vi "K6514_VISAQuery.vi"() -> ()   [LabVIEW 2024]
panel:
  out "read buffer":string
  in  "write buffer":string
  in  "VISA resource name":refnum<visa-resource-name>
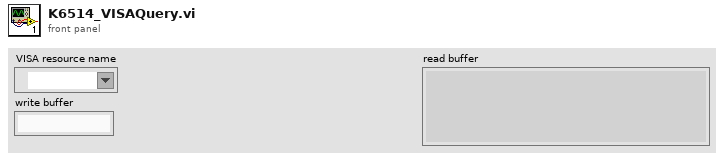
[diagram p1: front panel]
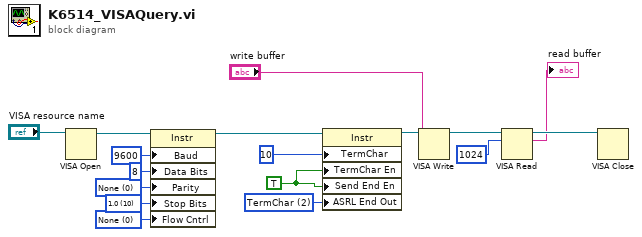
[diagram p0: block diagram]
diagram:
  w5 = u16 0 items=["None", "XON/XOFF", "RTS/CTS", "XON/XOFF & RTS/CTS", "DTR/DSR", "XON/XOFF & DTR/DSR"] ("Serial Settings:Flow Control")
  w6 = u16 10 items=["1.0"=10, "1.5"=15, "2.0"=20] ("Serial Settings:Stop Bits")
  w7 = u16 0 items=["None", "Odd", "Even", "Mark", "Space"] ("Serial Settings:Parity")
  w12 = u16 2 items=["None", "Last Bit", "TermChar", "Break"] ("Serial Settings:End Mode for Writes")
  w14 = TRUE
  n1 = VISA Open(VISA resource name="VISA resource name") -> (VISA resource name=w11:refnum<visa-resource-name>)  [unwired: 4 in, 1 out]
  n2 = property class="Instr"(reference=w11, "Baud"=u32 9600 ("Serial Settings:Baud Rate"), "Data Bits"=u16 8 ("Serial Settings:Data Bits"), "Parity"=w7, "Stop Bits"=w6, "Flow Cntrl"=w5) -> (reference out=w10:refnum<visa-resource-name>)  [unwired: 1 in, 1 out]
  n3 = property class="Instr"(reference=w10, "TermChar"=u8 10 ("Termination Character"), "TermChar En"=w14, "Send End En"=w14, "ASRL End Out"=w12) -> (reference out=w15:refnum<visa-resource-name>)  [unwired: 1 in, 1 out]
  n4 = VISA Write(VISA resource name=w15, write buffer="write buffer") -> (VISA resource name out=w4:refnum<visa-resource-name>)  [unwired: 1 in, 2 out]
  n5 = VISA Read(VISA resource name=w4, byte count=u32 1024) -> (VISA resource name out=w3:refnum<visa-resource-name>, read buffer=→"read buffer":string)  [unwired: 1 in, 2 out]
  n6 = VISA Close(VISA resource name=w3) -> ()  [unwired: 1 in, 1 out]
